vi "Driver Controller.vi"   [LabVIEW 2018]
uses:
  <vilib>/Rock Robotics/WPI/Joystick/WPI_JoystickDeviceEnum.ctl
  Driver Controller Global.vi
types:
  T1 = typedef "WPI_JoystickDeviceEnum.ctl" = enum16{"USB 0", "USB 1", "USB 2", "USB 3", "USB 4", "USB 5"}
  T2 = typedef "WPI_JoystickDevRef.ctl" = cluster{"Device":T1}
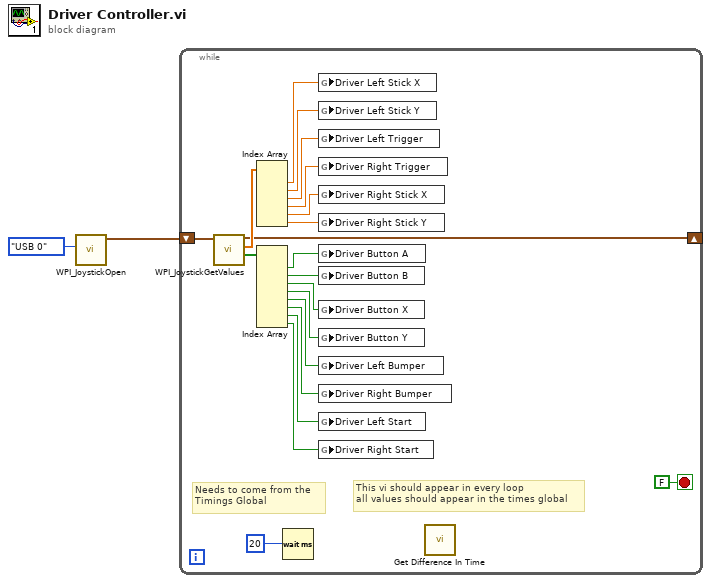
[diagram p0: block diagram]
diagram:
  n1 = call <vilib>:"WPI_JoystickOpen.vi"("JoystickDevice"=WPI_JoystickDeviceEnum."USB 0") -> ("JoystickDevRef"=w1:T2)  [unwired: 10 in]
  n2 = while {
    shift-right: [w5] -> _
    shift-left: w1 -> [w22]
    stop <- FALSE stop-if-true
    # "This vi should appear in every loop\nall values should appear in the times global"
    # "Needs to come from the\nTimings Global"
    n3 = call <vilib>:"WPI_JoystickGetValues.vi"("JoystickDevRef"=w22) -> ("Buttons"=w14:bool[], "Axes"=w21:dbl[], "JoystickDevRef"=w5:T2)  [unwired: 6 in, 2 out]
    n4 = Index Array(array=w21) -> (element #1=w20:dbl, element #2=w19:dbl, element #3=w18:dbl, element #4=w17:dbl, element #5=w16:dbl, element #6=w15:dbl)  [unwired: 6 in]
    n5 = Index Array(array=w14) -> (element #1=w13:bool, element #2=w12:bool, element #3=w11:bool, element #4=w10:bool, element #5=w9:bool, element #6=w8:bool, element #7=w7:bool, element #8=w6:bool)  [unwired: 8 in]
    n6 = Wait (ms)(milliseconds to wait=20) -> ()  [unwired: 1 out]
    n7 = global write "Driver Controller Global.vi" "Driver Left Stick X"(w20) -> ()
    n8 = global write "Driver Controller Global.vi" "Driver Left Stick Y"(w19) -> ()
    n9 = global write "Driver Controller Global.vi" "Driver Left Trigger"(w18) -> ()
    n10 = global write "Driver Controller Global.vi" "Driver Right Trigger"(w17) -> ()
    n11 = global write "Driver Controller Global.vi" "Driver Right Stick X"(w16) -> ()
    n12 = global write "Driver Controller Global.vi" "Driver Right Stick Y"(w15) -> ()
    n13 = global write "Driver Controller Global.vi" "Driver Button A"(w13) -> ()
    n14 = global write "Driver Controller Global.vi" "Driver Button B"(w12) -> ()
    n15 = global write "Driver Controller Global.vi" "Driver Button X"(w11) -> ()
    n16 = global write "Driver Controller Global.vi" "Driver Button Y"(w10) -> ()
    n17 = global write "Driver Controller Global.vi" "Driver Left Bumper"(w9) -> ()
    n18 = global write "Driver Controller Global.vi" "Driver Right Bumper"(w8) -> ()
    n19 = global write "Driver Controller Global.vi" "Driver Left Start"(w7) -> ()
    n20 = global write "Driver Controller Global.vi" "Driver Right Start"(w6) -> ()
    n21 = call "Get Difference In Time.vi"() -> ()  [unwired: 10 in, 2 out]
  }
